vi "MOSFET Test.vi"() -> ()   [LabVIEW 2017]
uses:
  <instrlib>/Keithley 2600 Series/Public/Channel.ctl
  <instrlib>/Keithley 2600 Series/Keithley 2600 Series.lvlib
panel:
  in  "stop":bool
  in  "Tab Control":T1(tab)
  in  "GateCluster DFC":T2={"Gate channel DFC"=0, "Operation Mode"=0, "GateStart DFC"=0.0, "GateStopDFC"=0.0, "GateStepDFC"=1.0, "GateComp DFC"=0.1, "GateStartUnit DFC"=1, "GateStopUnit DFC "=1, "GateStepUnit DFC"=1, "GateComplUnit DFC"=2} {"GateComplUnit DFC" items=["μA", "mA", "A"]; "GateStepUnit DFC" items=["mV", "V"]; "GateStopUnit DFC" items=["mV", "V"]; "GateStartUnit DFC" items=["mV", "V"]; "Gate channel DFC" items=["Channel A", "Channel B"]; "GateComp DFC" min=0.001 max=10.0 step=0.001; "GateStepDFC" min=-200.0 max=200.0 step=1.0 format="%#.3f"; "GateStopDFC" min=-200.0 max=200.0 step=1.0 format="%#.3f"; "GateStart DFC" min=-200.0 max=200.0 step=1.0 format="%#.3f"; "Operation Mode" items=["Voltage Step"]}
  in  "DrainCluster DFC":T3={"Drain "=0, "Operation Mode"=0, "DrainStart DFC"=0.0, "DrainStop DFC"=0.0, "DrainStep DFC"=1.0, "DrainComp DFC"=0.1, "DrainStartUnit DFC"=1, "DrainStopUnit  DFC"=1, "DrainStepUnit DFC"=1, "DrainCompUnit DFC"=2, "DrainDelayUnit DFC"=0, "DrainDelay DFC"=1.0} {"DrainDelay DFC" min=1.0 max=6000.0 step=1.0 format="%#.3f"; "DrainDelayUnit DFC" items=["ms", "s"]; "DrainCompUnit DFC" items=["μA", "mA", "A"]; "DrainStepUnit DFC" items=["mV", "V"]; "DrainStopUnit  DFC" items=["mV", "V"]; "DrainStartUnit DFC" items=["mV", "V"]; "Drain" items=["Channel A", "Channel B"]; "DrainComp DFC" min=0.1 max=1.0 step=0.001 format="%#.3f"; "DrainStep DFC" min=-200.0 max=200.0 step=1.0 format="%#.3f"; "DrainStop DFC" min=-200.0 max=200.0 step=1.0 format="%#.3f"; "DrainStart DFC" min=-200.0 max=200.0 step=1.0 format="%#.3f"; "Operation Mode" items=["Voltage Linear Sweep"]}
  out "Chart DFC":cluster{dbl[], dbl[]}[](graph)
  out "Sheet DFC":string[][](table) caption="Sheet"
  in  "GateCluster TV":T4={"Gate CHTV"=0, "Operation Mode"=0, "Start GateTV"=0.0, "Stop GateTV"=0.0, "Step GateTV"=0.0, "Comp GateTV"=0.0, "StartUnit GateTV"=1, "StopUnit GateTV"=1, "StepUnit GateTV"=1, "CompUnit GateTV"=2} {"CompUnit GateTV" items=["μA", "mA", "A"]; "StepUnit GateTV" items=["mV", "V"]; "StopUnit GateTV" items=["mV", "V"]; "StartUnit GateTV" items=["mV", "V"]; "Gate CHTV" items=["Channel A", "Channel B"]; "Operation Mode" items=["None", "Voltage Step", "Voltage bias "]}
  in  "DrainClusterTV":T5={"Drain CHTV"=0, "Operation Mode"=0, "Start DrainTV"=0.0, "Stop DrainTV"=0.0, "Step DrainTV"=0.0, "Comp DrainTV"=0.0, "StartUnit DrainTV"=1, "StopUnit DrainTV"=1, "StepUnit DrainTV"=1, "CompUnit DrainTV"=2} {"CompUnit DrainTV" items=["μA", "mA", "A"]; "StepUnit DrainTV" items=["mV", "V"]; "StopUnit DrainTV" items=["mV", "V"]; "StartUnit DrainTV" items=["mV", "V"]; "Drain CHTV" items=["Channel A", "Channel B"]; "Operation Mode" items=["None", "Voltage Step", ""]}
  out "Chart TV":cluster{dbl[], dbl[]}[](graph)
  out "Sheet TV":string[][](table) caption="Sheet"
  in  "GateCluster GL":T6={"Gate CHGL"=0, "Operation Mode"=0, "Start GateGL"=0.0, "Stop GateGL"=0.0, "Step GateGL"=0.0, "Comp GateGL"=0.0, "StartUnit GateGL"=1, "StopUnit GateGL"=1, "StepUnit GateGL"=1, "CompUnit GateGL"=2, "GateDelayUnit GL"=0, "GateDelay GL"=1.0} {"GateDelay GL" min=1.0 max=6000.0 step=1.0 format="%#.3f"; "GateDelayUnit GL" items=["ms", "s"]; "CompUnit GateGL" items=["μA", "mA", "A"]; "StepUnit GateGL" items=["mV", "V"]; "StopUnit GateGL" items=["mV", "V"]; "StartUnit GateGL" items=["mV", "V"]; "Gate CHGL" items=["Channel A", "Channel B"]; "Operation Mode" items=["Voltage Sweep"]}
  out "Chart GL":cluster{dbl[], dbl[]}[](graph)
  out "Sheet GL":string[][](table) caption="Sheet"
  in  "GateCluster Trans":T7={"G channeTR"=0, "Operation Mode"=0, "Start  GateTR"=0.0, "Stop GateTR"=0.0, "Step GateTR"=0.0, "Comp GateTR"=0.0, "StartUnit GateTR"=1, "StopUnit GateTR"=1, "StepUnit GateTR"=1, "CompUnit GateTR"=2, "GateDelayUnit TR"=0, "GateDelayTR"=1.0} {"GateDelayTR" min=1.0 max=6000.0 step=1.0 format="%#.3f"; "GateDelayUnit TR" items=["ms", "s"]; "CompUnit GateTR" items=["μA", "mA", "A"]; "StepUnit GateTR" items=["mV", "V"]; "StopUnit GateTR" items=["mV", "V"]; "StartUnit GateTR" items=["mV", "V"]; "G channeTR" items=["Channel A", "Channel B"]; "Operation Mode" items=["Voltage Step"]}
  in  "DrainCluster Trans":T8={"D channelTR"=0, "Operation Mode"=0, "Start DrainTR"=0.0, "Comp DrainTR"=0.0, "StartUnit DrainTR"=1, "CompUnit DrainTR"=2} {"CompUnit DrainTR" items=["μA", "mA", "A"]; "StartUnit DrainTR" items=["mV", "V"]; "D channelTR" items=["Channel A", "Channel B"]; "Operation Mode" items=["Voltage Bias"]}
  out "Chart TR":cluster{dbl[], dbl[]}[](graph)
  out "Sheet TR":string[][](table) caption="Sheet"
  in  "Save Button":bool
  in  "Stop Button":bool
  in  "OK Button":bool
  in  "Series 2600B":u16(ring)=5 items=["2602B  40V, 10A,100fA", "2604B  40V, 10A,100fA", "2612B  200V, 10A,100fA", "2614B  200V, 10A,100fA", "2634B  200V, 10A,1fA", "2636B  200V, 10A,0.1fA"]
  # "PRCBE  2600B -MOSFET Test"
  # "V"
  # "V"
  # "V"
  # "A"
  # "V"
  # "V"
  # "V"
  # "A"
  # "V"
  # "V"
  # "V"
  # "A"
  # "V"
  # "V"
  # "V"
  # "A"
  # "V"
  # "V"
  # "V"
  # "A"
  # "V"
  # "V"
  # "V"
  # "A"
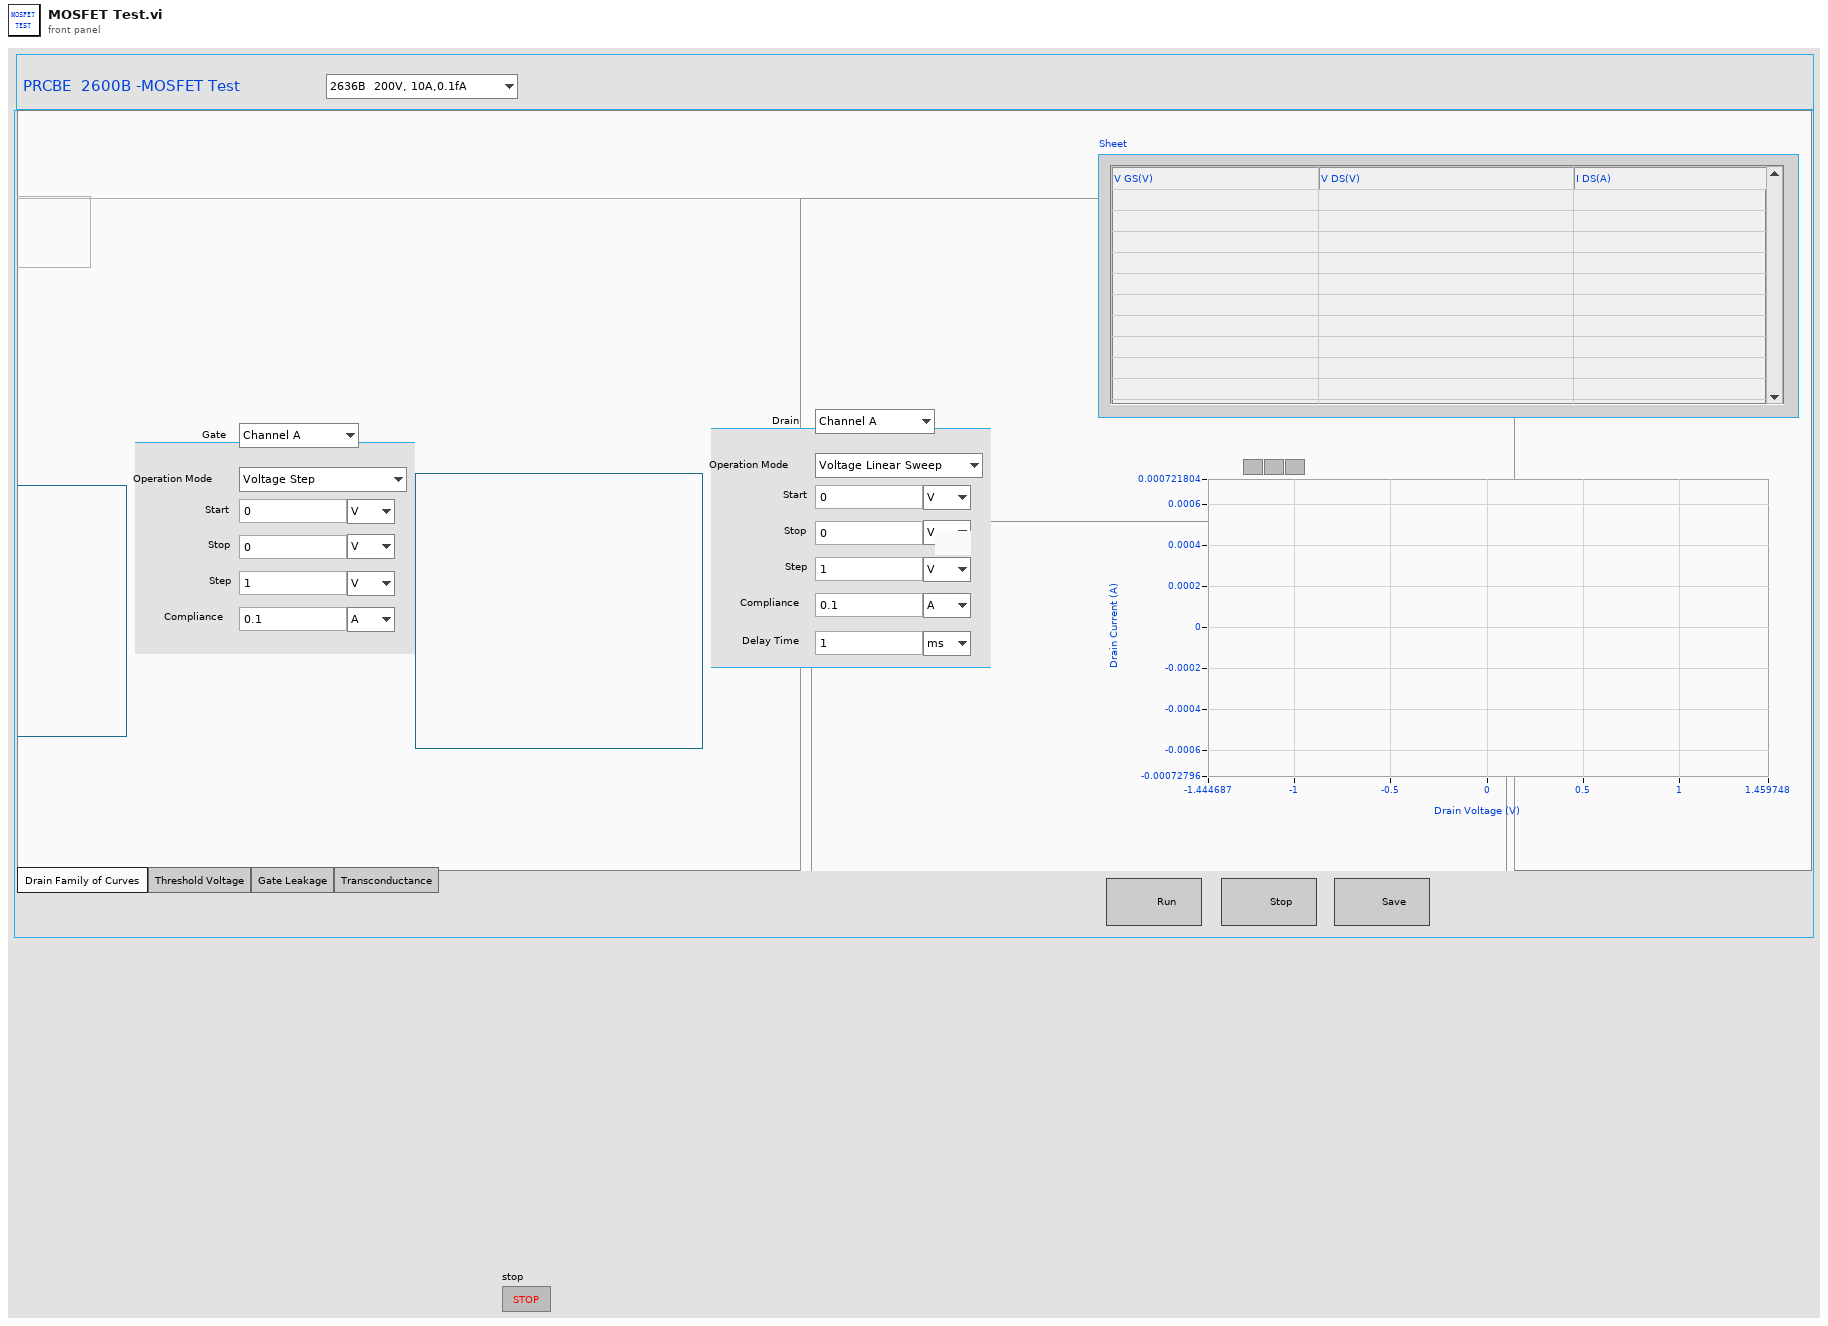
[diagram p1: front panel]
types:
  T1 = enum32{"Drain Family of Curves ", "Threshold Voltage", "Gate Leakage", "Transconductance"}
  T2 = cluster{"Gate channel DFC":u16, "Operation Mode":u16, "GateStart DFC":dbl, "GateStopDFC":dbl, "GateStepDFC":dbl, "GateComp DFC":dbl, "GateStartUnit DFC":u16, "GateStopUnit DFC ":u16, "GateStepUnit DFC":u16, "GateComplUnit DFC":u16}
  T3 = cluster{"Drain ":u16, "Operation Mode":u16, "DrainStart DFC":dbl, "DrainStop DFC":dbl, "DrainStep DFC":dbl, "DrainComp DFC":dbl, "DrainStartUnit DFC":u16, "DrainStopUnit  DFC":u16, "DrainStepUnit DFC":u16, "DrainCompUnit DFC":u16, "DrainDelayUnit DFC":u16, "DrainDelay DFC":dbl}
  T4 = cluster{"Gate CHTV":u16, "Operation Mode":u16, "Start GateTV":dbl, "Stop GateTV":dbl, "Step GateTV":dbl, "Comp GateTV":dbl, "StartUnit GateTV":u16, "StopUnit GateTV":u16, "StepUnit GateTV":u16, "CompUnit GateTV":u16}
  T5 = cluster{"Drain CHTV":u16, "Operation Mode":u16, "Start DrainTV":dbl, "Stop DrainTV":dbl, "Step DrainTV":dbl, "Comp DrainTV":dbl, "StartUnit DrainTV":u16, "StopUnit DrainTV":u16, "StepUnit DrainTV":u16, "CompUnit DrainTV":u16}
  T6 = cluster{"Gate CHGL":u16, "Operation Mode":u16, "Start GateGL":dbl, "Stop GateGL":dbl, "Step GateGL":dbl, "Comp GateGL":dbl, "StartUnit GateGL":u16, "StopUnit GateGL":u16, "StepUnit GateGL":u16, "CompUnit GateGL":u16, "GateDelayUnit GL":u16, "GateDelay GL":dbl}
  T7 = cluster{"G channeTR":u16, "Operation Mode":u16, "Start  GateTR":dbl, "Stop GateTR":dbl, "Step GateTR":dbl, "Comp GateTR":dbl, "StartUnit GateTR":u16, "StopUnit GateTR":u16, "StepUnit GateTR":u16, "CompUnit GateTR":u16, "GateDelayUnit TR":u16, "GateDelayTR":dbl}
  T8 = cluster{"D channelTR":u16, "Operation Mode":u16, "Start DrainTR":dbl, "Comp DrainTR":dbl, "StartUnit DrainTR":u16, "CompUnit DrainTR":u16}
  T9 = cluster{"Drain ":u16, "Operation Mode":u16, "DrainStart DFC":dbl, "DrainStop DFC":dbl, "DrainStep DFC":dbl, "DrainComp DFC":dbl, "DrainStartUnit DFC":u16, "DrainStopUnit  DFC":u16, "DrainStepUnit DFC":u16, "DrainCompUnit DFC":u16, "DrainDelay DFC":dbl, "DrainDelayUnit DFC":u16}
  T10 = typedef "Keithley 2600 Series.lvlib/Channel.ctl" = enum32{"Channel A", "Channel B"}
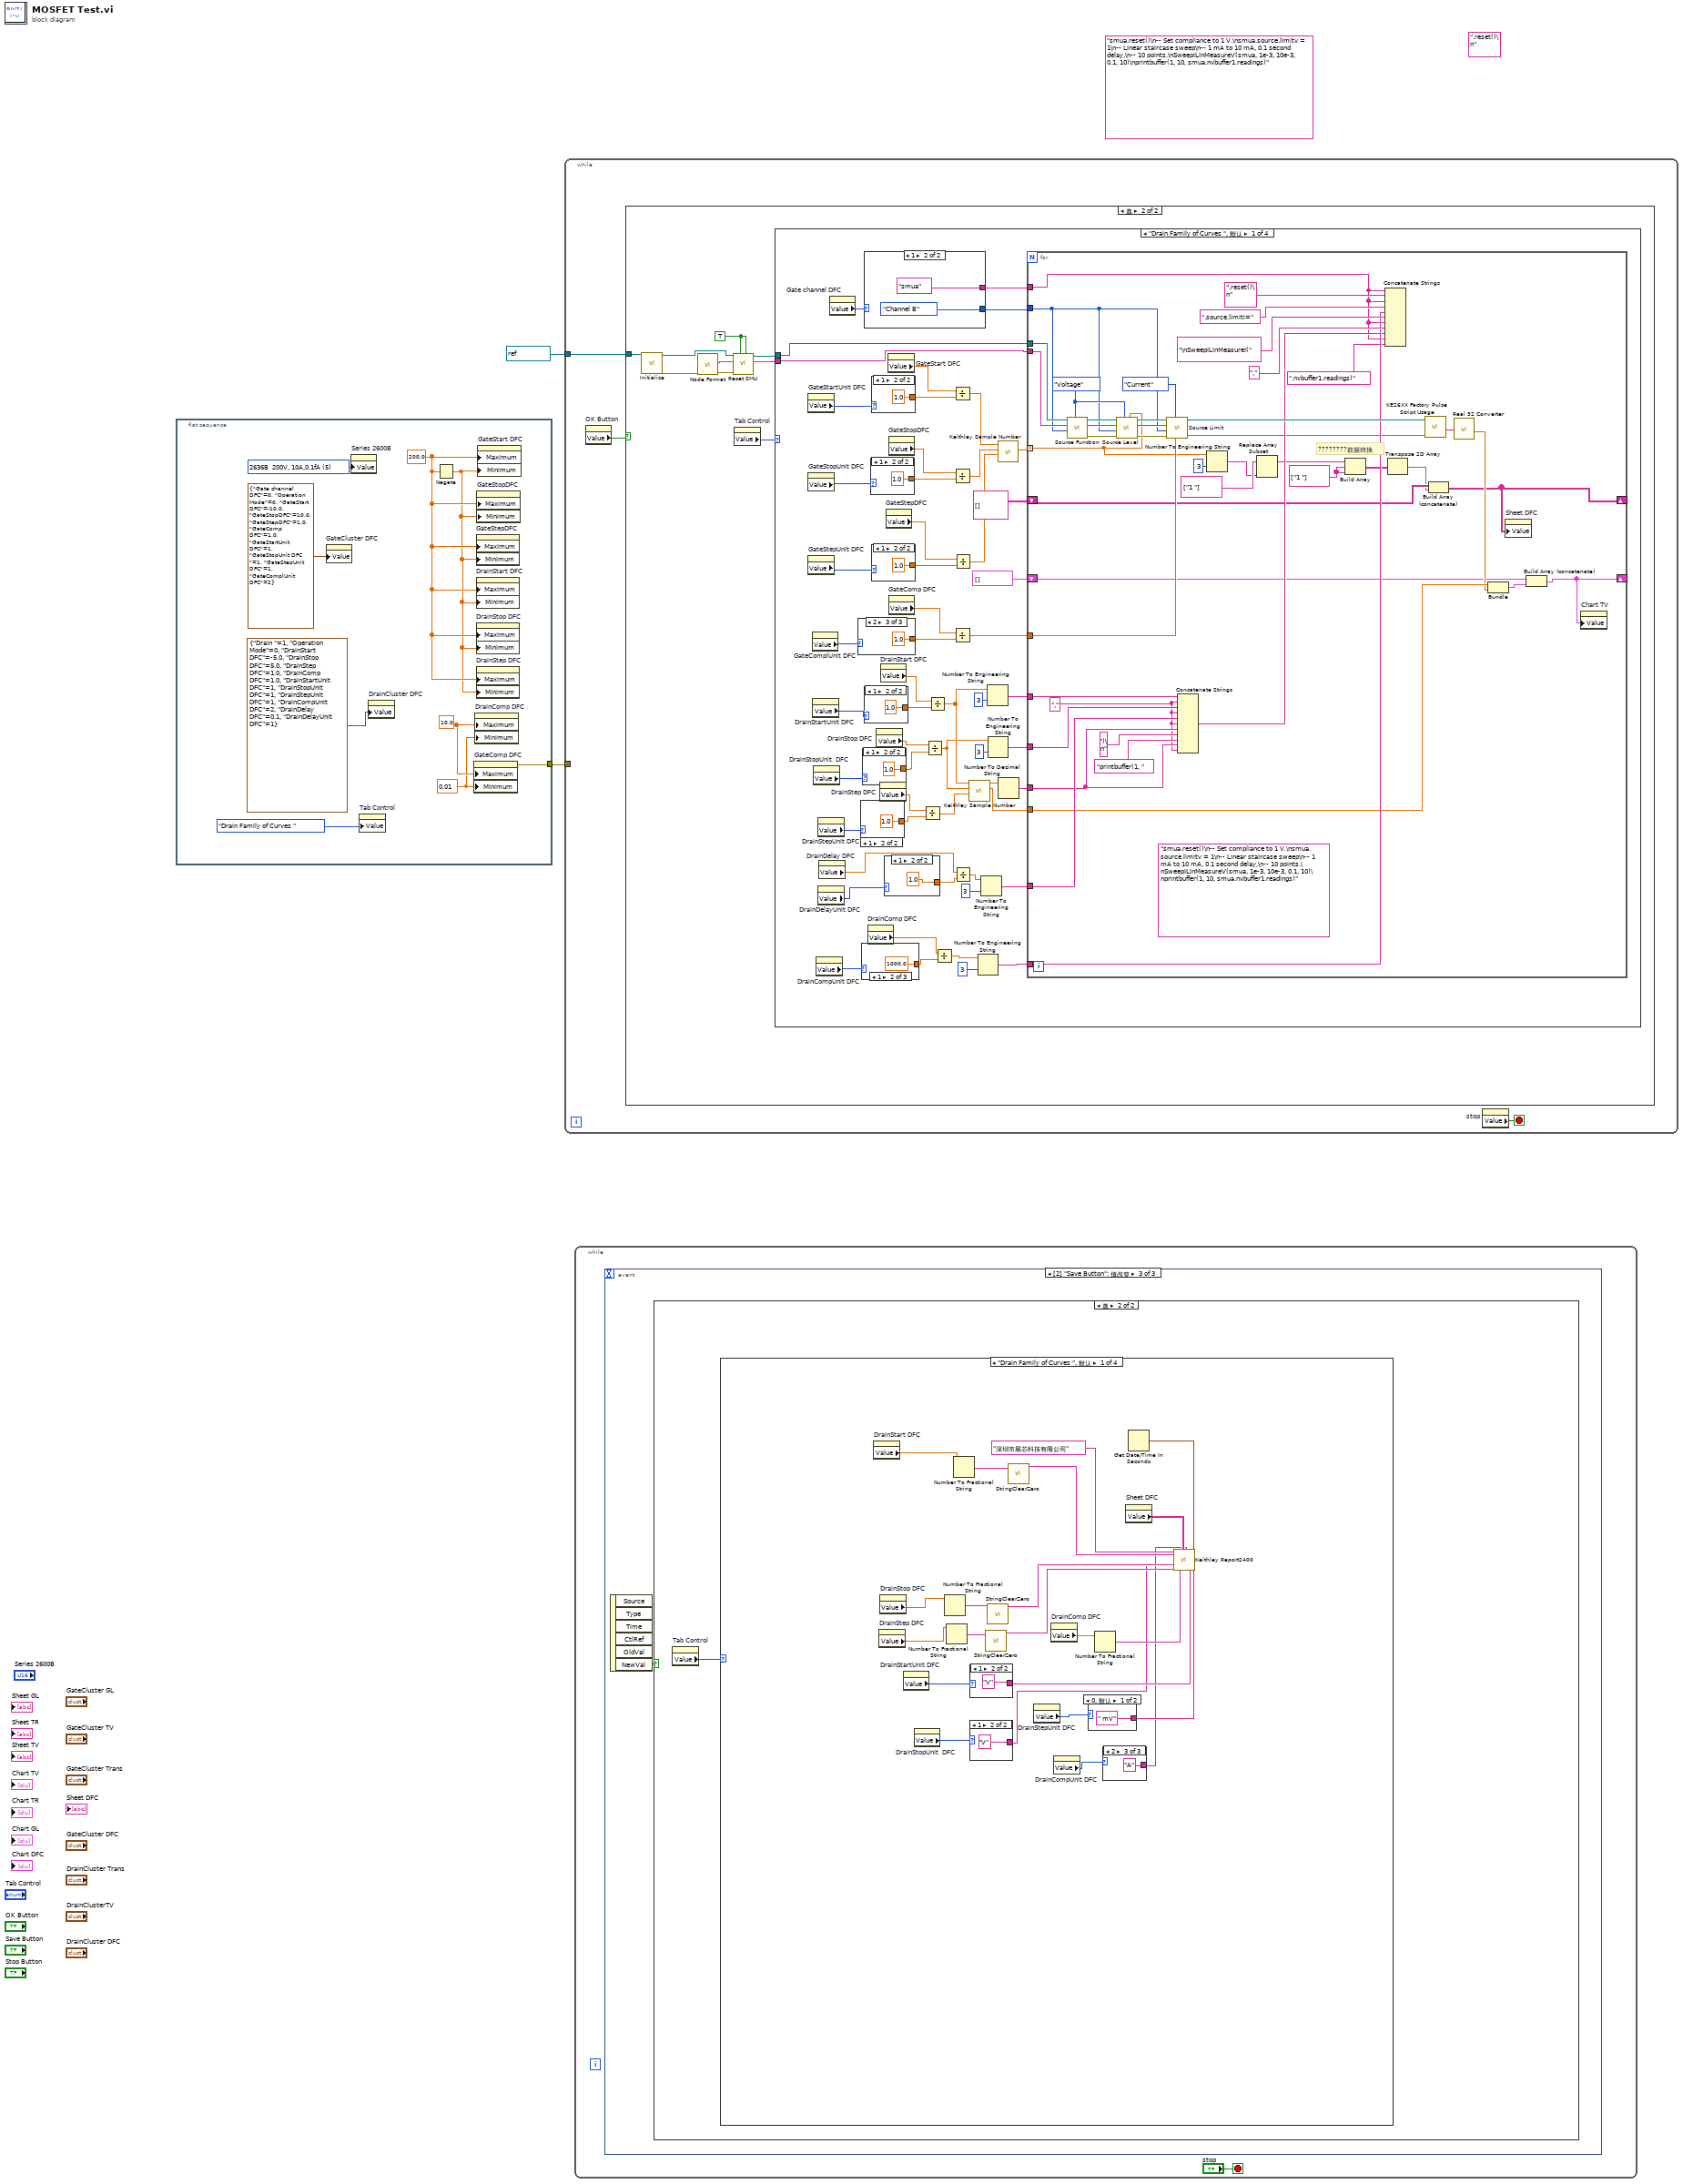
[diagram p0: block diagram]
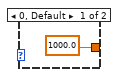
[diagram p3: hidden frame]
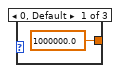
[diagram p4: hidden frame]
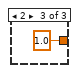
[diagram p5: hidden frame]
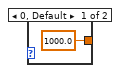
[diagram p6: hidden frame]
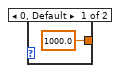
[diagram p7: hidden frame]
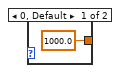
[diagram p8: hidden frame]
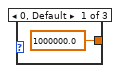
[diagram p9: hidden frame]
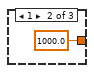
[diagram p10: hidden frame]
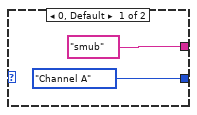
[diagram p11: hidden frame]
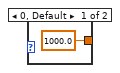
[diagram p12: hidden frame]
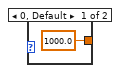
[diagram p13: hidden frame]
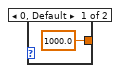
[diagram p14: hidden frame]
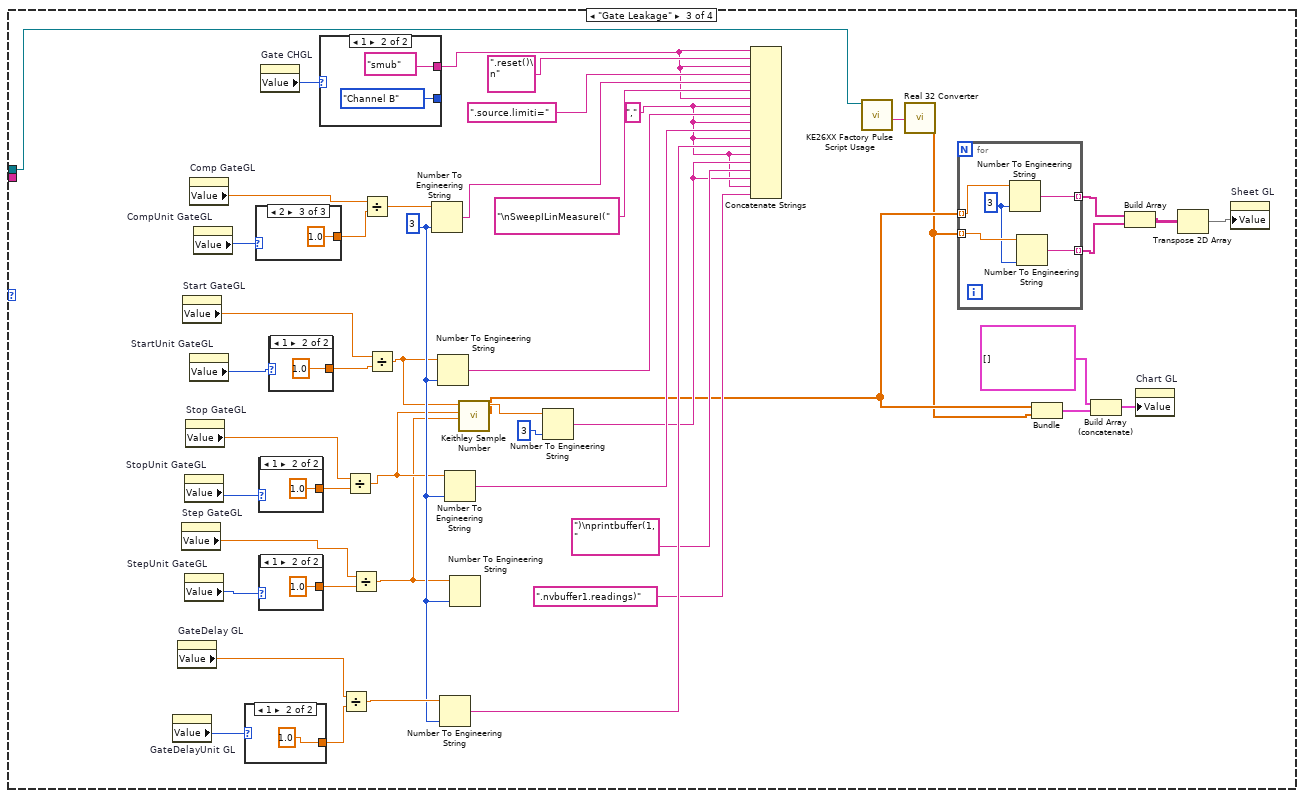
[diagram p16: hidden frame]
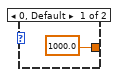
[diagram p17: hidden frame]
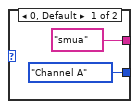
[diagram p18: hidden frame]
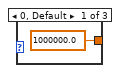
[diagram p19: hidden frame]
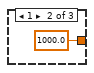
[diagram p20: hidden frame]
diagram:
  (unwired) ".reset()\n" ("string")
  (unwired) "smua.reset()\n-- Set compliance to 1 V.\nsmua.source.limitv = 1\n-- Linear staircase sweep\n-- 1 mA to 10 mA, 0.1 second delay,\n-- 10 points.\nSweepILinMeasureV(smua, 1e-3, 10e-3, 0.1, 10)\nprintbuffer(1, 10, smua.nvbuffer1.readings)" ("Script")
  n1 = flat-sequence {
    tunnel: [w3] -> w1
    frame #0 {
      w6 = 0.01 ("Data Entry Limits:Minimum")
      w7 = 10.0 ("Data Entry Limits:Maximum")
      w9 = 200.0 ("Data Entry Limits:Maximum")
      w11 = u16 5 items=["2602B  40V, 10A,100fA", "2604B  40V, 10A,100fA", "2612B  200V, 10A,100fA", "2614B  200V, 10A,100fA", "2634B  200V, 10A,1fA", "2636B  200V, 10A,0.1fA"] ("Series 2600B")
      n2 = property on="GateCluster DFC" class="Clust (严格)"("Value"=T2 {"Gate channel DFC"=0, "Operation Mode"=0, "GateStart DFC"=-10.0, "GateStopDFC"=10.0, "GateStepDFC"=1.0, "GateComp DFC"=1.0, "GateStartUnit DFC"=1, "GateStopUnit DFC "=1, "GateStepUnit DFC"=1, "GateComplUnit DFC"=2} ("GateCluster DFC")) -> ()  [unwired: 2 in, 2 out]
      n3 = property on="Series 2600B" class="Ring (严格)"("Value"=w11) -> ()  [unwired: 2 in, 2 out]
      n4 = property on="Tab Control" class="TabCtl (严格)"("Value"=T1."Drain Family of Curves " ("Tab Control")) -> ()  [unwired: 2 in, 2 out]
      n5 = property on="DrainCluster DFC" class="Clust (严格)"("Value"=T9 {"Drain "=1, "Operation Mode"=0, "DrainStart DFC"=-5.0, "DrainStop DFC"=5.0, "DrainStep DFC"=1.0, "DrainComp DFC"=1.0, "DrainStartUnit DFC"=1, "DrainStopUnit  DFC"=1, "DrainStepUnit DFC"=1, "DrainCompUnit DFC"=2, "DrainDelay DFC"=0.1, "DrainDelayUnit DFC"=1} ("DrainCluster DFC")) -> ()  [unwired: 2 in, 2 out]
      n6 = Negate(x=w9) -> (-x=w8:dbl)
      n7 = property on="GateComp DFC" class="DigNum (严格)"("Maximum"=w7, "Minimum"=w6) -> (error out=w3:errorcluster)  [unwired: 2 in, 1 out]
      n8 = property on="DrainComp DFC" class="DigNum (严格)"("Maximum"=w7, "Minimum"=w6) -> ()  [unwired: 2 in, 2 out]
      n9 = property on="GateStepDFC" class="DigNum (严格)"("Maximum"=w9, "Minimum"=w8) -> ()  [unwired: 2 in, 2 out]
      n10 = property on="DrainStart DFC" class="DigNum (严格)"("Maximum"=w9, "Minimum"=w8) -> ()  [unwired: 2 in, 2 out]
      n11 = property on="DrainStop DFC" class="DigNum (严格)"("Maximum"=w9, "Minimum"=w8) -> ()  [unwired: 2 in, 2 out]
      n12 = property on="DrainStep DFC" class="DigNum (严格)"("Maximum"=w9, "Minimum"=w8) -> ()  [unwired: 2 in, 2 out]
      n13 = property on="GateStopDFC" class="DigNum (严格)"("Maximum"=w9, "Minimum"=w8) -> ()  [unwired: 2 in, 2 out]
      n14 = property on="GateStart DFC" class="DigNum (严格)"("Maximum"=w9, "Minimum"=w8) -> ()  [unwired: 2 in, 2 out]
    }
  }
  n15 = while {
    tunnel: refnum<visa-resource-name> "COM1" ("VISA resource name") -> [w12]
    tunnel: w1 -> [_]
    stop <- w14 stop-if-true
    n16 = property on="OK Button" class="Bool (严格)"() -> ("Value"=w13:bool)  [unwired: 2 in, 2 out]
    n17 = case shown="真" w13 {
      tunnel: w12 -> [_ w22]
      frame False {
      }
      frame True {
        w17 = TRUE ("SMU A (No)")
        n18 = call <instrlib>:"Initialize.vi"("VISA resource name"=w22) -> ("error out"=w21:errorcluster, "VISA resource name out"=w20:refnum<visa-resource-name>)  [unwired: 4 in, 5 out]
        n19 = call <instrlib>:"Node Format.vi"("error in"=w21) -> ("error out"=w18:errorcluster, "Formatted Node"=w19:string)  [unwired: 1 in, 8 out]
        n20 = call <instrlib>:"Reset SMU.vi"("SMU B (No)"=w17, "SMU A (No)"=w17, "error in (no error)"=w18, "Node In"=w19, "VISA resource name"=w20) -> ("Node Out"=w15:string, "VISA resource name out"=w16:refnum<visa-resource-name>)  [unwired: 5 out]
        n21 = property on="Tab Control" class="TabCtl (严格)"() -> ("Value"=w23:T1)  [unwired: 2 in, 2 out]
        n22 = case shown="\"Drain Family of Curves \", 默认" w23 {
          tunnel: w16 -> [w65 _ w176 w227]
          tunnel: w15 -> [w63 _ _ w223]
          frame "Drain Family of Curves ", Default {
            n23 = property on="GateStartUnit DFC" class="Ring (严格)"() -> ("Value"=w78:u16)  [unwired: 2 in, 2 out]
            n24 = property on="GateStopUnit DFC" class="Ring (严格)"() -> ("Value"=w75:u16)  [unwired: 2 in, 2 out]
            n25 = property on="GateStepUnit DFC" class="Ring (严格)"() -> ("Value"=w72:u16)  [unwired: 2 in, 2 out]
            n26 = property on="GateComplUnit DFC" class="Ring (严格)"() -> ("Value"=w61:u16)  [unwired: 2 in, 2 out]
            n27 = property on="DrainStartUnit DFC" class="Ring (严格)"() -> ("Value"=w55:u16)  [unwired: 2 in, 2 out]
            n28 = property on="DrainStopUnit  DFC" class="Ring (严格)"() -> ("Value"=w52:u16)  [unwired: 2 in, 2 out]
            n29 = property on="DrainCompUnit DFC" class="Ring (严格)"() -> ("Value"=w43:u16)  [unwired: 2 in, 2 out]
            n30 = property on="DrainStepUnit DFC" class="Ring (严格)"() -> ("Value"=w51:u16)  [unwired: 2 in, 2 out]
            n31 = property on="DrainDelayUnit DFC" class="Ring (严格)"() -> ("Value"=w29:u16)  [unwired: 2 in, 2 out]
            n32 = property on="DrainDelay DFC" class="DigNum (严格)"() -> ("Value"=w33:dbl)  [unwired: 2 in, 2 out]
            n33 = property on="Gate channel DFC" class="Ring (严格)"() -> ("Value"=w64:u16)  [unwired: 2 in, 2 out]
            n34 = case shown="2" w61 {
              tunnel: [1000000.0 ("Value") 1000.0 ("Value") 1.0 ("Value")] -> w60
              frame 0, Default {
              }
              frame 1 {
              }
              frame 2 {
              }
            }
            n35 = case shown="1" w51 {
              tunnel: [1000.0 ("Value") 1.0 ("Value")] -> w48
              frame 0, Default {
              }
              frame 1 {
              }
            }
            n36 = case shown="1" w43 {
              tunnel: [1000000.0 ("Value") 1000.0 ("Value") 1.0 ("Value")] -> w45
              frame 0, Default {
              }
              frame 1 {
              }
              frame 2 {
              }
            }
            n37 = case shown="1" w52 {
              tunnel: [1000.0 ("Value") 1.0 ("Value")] -> w49
              frame 0, Default {
              }
              frame 1 {
              }
            }
            n38 = case shown="1" w64 {
              tunnel: [Channel."Channel A" ("Channel (Channel A)") Channel."Channel B" ("Channel (Channel A)")] -> w62
              tunnel: ["smub" ("Script") "smua" ("Script")] -> w57
              frame 0, Default {
              }
              frame 1 {
              }
            }
            n39 = case shown="1" w55 {
              tunnel: [1000.0 ("Value") 1.0 ("Value")] -> w56
              frame 0, Default {
              }
              frame 1 {
              }
            }
            n40 = property on="DrainComp DFC" class="DigNum (严格)"() -> ("Value"=w44:dbl)  [unwired: 2 in, 2 out]
            n41 = case shown="1" w75 {
              tunnel: [1000.0 ("Value") 1.0 ("Value")] -> w73
              frame 0, Default {
              }
              frame 1 {
              }
            }
            n42 = case shown="1" w78 {
              tunnel: [1000.0 ("Value") 1.0 ("Value")] -> w77
              frame 0, Default {
              }
              frame 1 {
              }
            }
            n43 = case shown="1" w72 {
              tunnel: [1000.0 ("Value") 1.0 ("Value")] -> w71
              frame 0, Default {
              }
              frame 1 {
              }
            }
            n44 = property on="DrainStop DFC" class="DigNum (严格)"() -> ("Value"=w53:dbl)  [unwired: 2 in, 2 out]
            n45 = property on="DrainStep DFC" class="DigNum (严格)"() -> ("Value"=w50:dbl)  [unwired: 2 in, 2 out]
            n46 = property on="DrainStart DFC" class="DigNum (严格)"() -> ("Value"=w54:dbl)  [unwired: 2 in, 2 out]
            n47 = case shown="1" w29 {
              tunnel: [1000.0 ("Value") 1.0 ("Value")] -> w32
              frame 0, Default {
              }
              frame 1 {
              }
            }
            n48 = property on="GateStepDFC" class="DigNum (严格)"() -> ("Value"=w70:dbl)  [unwired: 2 in, 2 out]
            n49 = property on="GateStart DFC" class="DigNum (严格)"() -> ("Value"=w76:dbl)  [unwired: 2 in, 2 out]
            n50 = property on="GateStopDFC" class="DigNum (严格)"() -> ("Value"=w74:dbl)  [unwired: 2 in, 2 out]
            n51 = property on="GateComp DFC" class="DigNum (严格)"() -> ("Value"=w59:dbl)  [unwired: 2 in, 2 out]
            n52 = Divide(x=w50, y=w48) -> (x/y=w47:dbl)
            n53 = Divide(x=w53, y=w49) -> (x/y=w27:dbl)
            n54 = Divide(x=w54, y=w56) -> (x/y=w37:dbl)
            n55 = Divide(x=w44, y=w45) -> (x/y=w41:dbl)
            n56 = Divide(x=w76, y=w77) -> (x/y=w69:dbl)
            n57 = Divide(x=w74, y=w73) -> (x/y=w68:dbl)
            n58 = Divide(x=w59, y=w60) -> (x/y=w58:dbl)
            n59 = Divide(x=w70, y=w71) -> (x/y=w67:dbl)
            n60 = Divide(x=w33, y=w32) -> (x/y=w30:dbl)
            n61 = call "Keithley Sample Number.vi"("Step"=w47, "Stop"=w27, "Start"=w37) -> ("Array"=w26:dbl[], "pointnumber"=w46:dbl)  [unwired: 7 in]
            n62 = Number To Engineering String(2:i16 3 ("precision (6)"), 4:w41) -> (0:w40:string)  [unwired: 2 in]
            n63 = Number To Engineering String(2:i16 3 ("precision (6)"), 4:w30) -> (0:w28:string)  [unwired: 2 in]
            n64 = Number To Engineering String(2:i16 3 ("precision (6)"), 4:w37) -> (0:w34:string)  [unwired: 2 in]
            n65 = Number To Engineering String(2:i16 3 ("precision (6)"), 4:w27) -> (0:w35:string)  [unwired: 2 in]
            n66 = call "Keithley Sample Number.vi"("Step"=w67, "Stop"=w68, "Start"=w69) -> ("Array"=w66:dbl[])  [unwired: 7 in, 1 out]
            n67 = Number To Decimal String(number=w46) -> (decimal integer string=w39:string)  [unwired: 1 in]
            n68 = for {
              tunnel: w66 -> [w105] mode=indexing
              tunnel: w65 -> [w137]
              tunnel: w63 -> [w136]
              tunnel: w62 -> [w132]
              tunnel: w58 -> [w127]
              tunnel: w57 -> [w116]
              tunnel: w40 -> [w124]
              tunnel: w39 -> [w118]
              tunnel: w35 -> [w122]
              tunnel: w34 -> [w123]
              tunnel: w28 -> [w121]
              tunnel: w26 -> [w111]
              shift-right: [w107] -> _
              shift-left: cluster{dbl[], dbl[]}[] [] ("Chart TV") -> [w109]
              shift-right: [w97] -> _
              shift-left: string[][] [] ("Sheet DFC") -> [w103]
              w104 = string[] ["1 "]
              (unwired) "smua.reset()\n-- Set compliance to 1 V.\nsmua.source.limitv = 1\n-- Linear staircase sweep\n-- 1 mA to 10 mA, 0.1 second delay,\n-- 10 points.\nSweepILinMeasureV(smua, 1e-3, 10e-3, 0.1, 10)\nprintbuffer(1, 10, smua.nvbuffer1.readings)" ("Script")
              w115 = "," ("string")
              w135 = enum32{"Current", "Voltage"}."Voltage" ("Function (Current)")
              # "????????数据转换"
              n69 = call <instrlib>:"Source Function.vi"("Function (Current)"=w135, "Channel (Channel A)"=w132, "Node In"=w136, "VISA resource name"=w137) -> ("error out"=w134:errorcluster, "Node Out"=w138:string, "VISA resource name out"=w139:refnum<visa-resource-name>)  [unwired: 1 in, 4 out]
              n70 = call <instrlib>:"Source Level.vi"("Level (0.000)"=w105, "Function (Current)"=w135, "error in (no error)"=w134, "Channel (Channel A)"=w132, "Node In"=w138, "VISA resource name"=w139) -> ("error out"=w133:errorcluster, "Node Out"=w141:string, "VISA resource name out"=w140:refnum<visa-resource-name>)  [unwired: 3 out]
              n71 = call <instrlib>:"Source Limit.vi"("Limit (0.000)"=w127, "Function (Current)"=enum32{"Current", "Voltage"}."Current", "error in (no error)"=w133, "Channel (Channel A)"=w132, "Node In"=w141, "VISA resource name"=w140) -> ("error out"=w113:errorcluster, "VISA resource name out"=w130:refnum<visa-resource-name>)  [unwired: 4 out]
              n72 = Concatenate Strings(w123, w115, w122, w115, w121, w115, w118, ")\n" ("string"), "printbuffer(1, " ("string"), w118, w115) -> (w117:string)
              n73 = Number To Engineering String(2:i16 3 ("precision (6)"), 4:w105) -> (0:w101:string)  [unwired: 2 in]
              n74 = Replace Array Subset(array=string[] ["1 "], new element=w101) -> (w100:string[])  [unwired: 1 in]
              n75 = Build Array(w100, w104, w104) -> (w99:string[][])
              n76 = Concatenate Strings(w116, ".reset()\n" ("string"), w116, ".source.limiti=" ("string"), w124, "\nSweepILinMeasureI(" ("string"), w116, "," ("string"), w117, w116, ".nvbuffer1.readings)" ("string")) -> ()  [unwired: 1 out]
              n77 = Transpose 2D Array(2D array=w99) -> (transposed array=w98:string[][])
              n78 = call <instrlib>:"KE26XX Factory Pulse Script Usage.vi"("error in"=w113, "VISA resource name"=w130) -> ("Buffer Data"=w112:string)  [unwired: 8 in, 1 out]
              n79 = Build Array (concatenate)(w103, w98) -> (w97:string[][])
              n80 = call <instrlib>:"Real 32 Converter.vi"("Data In"=w112) -> ("Data Array Out"=w110:sgl[])  [unwired: 10 in]
              n81 = Bundle("Array"=w111, "Data Array Out"=w110) -> (w108:cluster{"Array":dbl[], "Data Array Out":sgl[]})  [unwired: 1 in]
              n82 = property on="Sheet DFC" class="Tbl (严格)"("Value"=w97) -> ()  [unwired: 2 in, 2 out]
              n83 = Build Array (concatenate)(w109, w108) -> (w107:cluster{"Array":dbl[], "Data Array Out":dbl[]}[])
              n84 = property on="Chart TV" class="XYGraph (严格)"("Value"=w107) -> ()  [unwired: 2 in, 2 out]
            }
          }
          frame "Threshold Voltage" {
          }
          frame "Gate Leakage" {
            w158 = "," ("string")
            w174 = i16 3 ("precision (6)")
            n85 = property on="GateDelayUnit GL" class="Ring (严格)"() -> ("Value"=w173:u16)  [unwired: 2 in, 2 out]
            n86 = property on="GateDelay GL" class="DigNum (严格)"() -> ("Value"=w171:dbl)  [unwired: 2 in, 2 out]
            n87 = property on="Step GateGL" class="DigNum (严格)"() -> ("Value"=w187:dbl)  [unwired: 2 in, 2 out]
            n88 = property on="Start GateGL" class="DigNum (严格)"() -> ("Value"=w193:dbl)  [unwired: 2 in, 2 out]
            n89 = property on="StopUnit GateGL" class="Ring (严格)"() -> ("Value"=w189:u16)  [unwired: 2 in, 2 out]
            n90 = property on="StepUnit GateGL" class="Ring (严格)"() -> ("Value"=w186:u16)  [unwired: 2 in, 2 out]
            n91 = property on="Stop GateGL" class="DigNum (严格)"() -> ("Value"=w190:dbl)  [unwired: 2 in, 2 out]
            n92 = property on="Comp GateGL" class="DigNum (严格)"() -> ("Value"=w184:dbl)  [unwired: 2 in, 2 out]
            n93 = property on="StartUnit GateGL" class="Ring (严格)"() -> ("Value"=w194:u16)  [unwired: 2 in, 2 out]
            n94 = property on="CompUnit GateGL" class="Ring (严格)"() -> ("Value"=w183:u16)  [unwired: 2 in, 2 out]
            n95 = case shown="1" w173 {
              tunnel: [1000.0 ("Value") 1.0 ("Value")] -> w172
              frame 0, Default {
              }
              frame 1 {
              }
            }
            n96 = case shown="2" w183 {
              tunnel: [1000000.0 ("Value") 1000.0 ("Value") 1.0 ("Value")] -> w185
              frame 0, Default {
              }
              frame 1 {
              }
              frame 2 {
              }
            }
            n97 = case shown="1" w189 {
              tunnel: [1000.0 ("Value") 1.0 ("Value")] -> w191
              frame 0, Default {
              }
              frame 1 {
              }
            }
            n98 = case shown="1" w186 {
              tunnel: [1000.0 ("Value") 1.0 ("Value")] -> w188
              frame 0, Default {
              }
              frame 1 {
              }
            }
            n99 = property on="Gate CHGL" class="Ring (严格)"() -> ("Value"=w182:u16)  [unwired: 2 in, 2 out]
            n100 = case shown="1" w194 {
              tunnel: [1000.0 ("Value") 1.0 ("Value")] -> w192
              frame 0, Default {
              }
              frame 1 {
              }
            }
            n101 = case shown="1" w182 {
              tunnel: [Channel."Channel A" ("Channel (Channel A)") Channel."Channel B" ("Channel (Channel A)")] -> _
              tunnel: ["smua" ("Script") "smub" ("Script")] -> w166
              frame 0, Default {
              }
              frame 1 {
              }
            }
            n102 = Divide(x=w171, y=w172) -> (x/y=w175:dbl)
            n103 = Divide(x=w190, y=w191) -> (x/y=w169:dbl)
            n104 = Divide(x=w187, y=w188) -> (x/y=w168:dbl)
            n105 = Divide(x=w184, y=w185) -> (x/y=w178:dbl)
            n106 = Divide(x=w193, y=w192) -> (x/y=w170:dbl)
            n107 = Number To Engineering String(2:w174, 4:w178) -> (0:w177:string)  [unwired: 2 in]
            n108 = Number To Engineering String(2:w174, 4:w170) -> (0:w165:string)  [unwired: 2 in]
            n109 = Number To Engineering String(2:w174, 4:w175) -> (0:w163:string)  [unwired: 2 in]
            n110 = Number To Engineering String(2:w174, 4:w169) -> (0:w164:string)  [unwired: 2 in]
            n111 = Number To Engineering String(2:w174, 4:w168) -> ()  [unwired: 2 in, 1 out]
            n112 = call "Keithley Sample Number.vi"("Step"=w168, "Stop"=w169, "Start"=w170) -> ("Array"=w152:dbl[], "pointnumber"=w161:dbl)  [unwired: 7 in]
            n113 = Number To Engineering String(2:i16 3 ("precision (6)"), 4:w161) -> (0:w159:string)  [unwired: 2 in]
            n114 = Concatenate Strings(w166, ".reset()\n" ("string"), w166, ".source.limiti=" ("string"), w177, "\nSweepILinMeasureI(" ("string"), w166, w158, w165, w158, w164, w158, w163, w158, w159, ")\nprintbuffer(1, " ("string"), w159, w158, ".nvbuffer1.readings)" ("string")) -> ()  [unwired: 1 out]
            n115 = call <instrlib>:"KE26XX Factory Pulse Script Usage.vi"("VISA resource name"=w176) -> ("Buffer Data"=w181:string)  [unwired: 9 in, 1 out]
            n116 = call <instrlib>:"Real 32 Converter.vi"("Data In"=w181) -> ("Data Array Out"=w151:sgl[])  [unwired: 10 in]
            n117 = for {
              tunnel: w152 -> [w199] mode=indexing
              tunnel: w151 -> [w197] mode=indexing
              tunnel: [w198] -> w150 mode=indexing
              tunnel: [w195] -> w149 mode=indexing
              w196 = i16 3 ("precision (6)")
              n118 = Number To Engineering String(2:w196, 4:w199) -> (0:w198:string)  [unwired: 2 in]
              n119 = Number To Engineering String(2:w196, 4:w197) -> (0:w195:string)  [unwired: 2 in]
            }
            n120 = Bundle("Array"=w152, "Data Array Out"=w151) -> (w155:cluster{"Array":dbl[], "Data Array Out":sgl[]})  [unwired: 1 in]
            n121 = Build Array (concatenate)(cluster{dbl[], dbl[]}[] [] ("Chart GL"), w155) -> (w154:cluster{"Array":dbl[], "Data Array Out":dbl[]}[])
            n122 = Build Array(w150, w149) -> (w153:string[][])
            n123 = property on="Chart GL" class="XYGraph (严格)"("Value"=w154) -> ()  [unwired: 2 in, 2 out]
            n124 = Transpose 2D Array(2D array=w153) -> (transposed array=w148:string[][])
            n125 = property on="Sheet GL" class="Tbl (严格)"("Value"=w148) -> ()  [unwired: 2 in, 2 out]
          }
          frame "Transconductance" {
            w231 = enum32{"Current", "Voltage"}."Voltage" ("Function (Current)")
            w247 = "," ("string")
            w263 = i16 3 ("precision (6)")
            # "??/????数据转换确认"
            n126 = property on="GateDelayTR" class="DigNum (严格)"() -> ("Value"=w260:dbl)  [unwired: 2 in, 2 out]
            n127 = property on="GateDelayUnit TR" class="Ring (严格)"() -> ("Value"=w262:u16)  [unwired: 2 in, 2 out]
            n128 = property on="Step GateTR" class="DigNum (严格)"() -> ("Value"=w274:dbl)  [unwired: 2 in, 2 out]
            n129 = property on="Stop GateTR" class="DigNum (严格)"() -> ("Value"=w277:dbl)  [unwired: 2 in, 2 out]
            n130 = property on="StopUnit GateTR" class="Ring (严格)"() -> ("Value"=w276:u16)  [unwired: 2 in, 2 out]
            n131 = property on="StepUnit GateTR" class="Ring (严格)"() -> ("Value"=w273:u16)  [unwired: 2 in, 2 out]
            n132 = property on="StartUnit GateTR" class="Ring (严格)"() -> ("Value"=w281:u16)  [unwired: 2 in, 2 out]
            n133 = property on="Start  GateTR" class="DigNum (严格)"() -> ("Value"=w280:dbl)  [unwired: 2 in, 2 out]
            n134 = property on="Comp GateTR" class="DigNum (严格)"() -> ("Value"=w271:dbl)  [unwired: 2 in, 2 out]
            n135 = property on="CompUnit GateTR" class="Ring (严格)"() -> ("Value"=w270:u16)  [unwired: 2 in, 2 out]
            n136 = property on="CompUnit DrainTR" class="Ring (严格)"() -> ("Value"=w219:u16)  [unwired: 2 in, 2 out]
            n137 = property on="G channeTR" class="Ring (严格)"() -> ("Value"=w245:u16)  [unwired: 2 in, 2 out]
            n138 = property on="Comp DrainTR" class="DigNum (严格)"() -> ("Value"=w218:dbl)  [unwired: 2 in, 2 out]
            n139 = property on="StartUnit DrainTR" class="Ring (严格)"() -> ("Value"=w216:u16)  [unwired: 2 in, 2 out]
            n140 = property on="Start DrainTR" class="DigNum (严格)"() -> ("Value"=w222:dbl)  [unwired: 2 in, 2 out]
            n141 = case shown="1" w262 {
              tunnel: [1000.0 ("Value") 1.0 ("Value")] -> w261
              frame 0, Default {
              }
              frame 1 {
              }
            }
            n142 = case shown="2" w270 {
              tunnel: [1000000.0 ("Value") 1000.0 ("Value") 1.0 ("Value")] -> w272
              frame 0, Default {
              }
              frame 1 {
              }
              frame 2 {
              }
            }
            n143 = case shown="1" w276 {
              tunnel: [1000.0 ("Value") 1.0 ("Value")] -> w278
              frame 0, Default {
              }
              frame 1 {
              }
            }
            n144 = case shown="1" w273 {
              tunnel: [1000.0 ("Value") 1.0 ("Value")] -> w275
              frame 0, Default {
              }
              frame 1 {
              }
            }
            n145 = case shown="1" w281 {
              tunnel: [1000.0 ("Value") 1.0 ("Value")] -> w279
              frame 0, Default {
              }
              frame 1 {
              }
            }
            n146 = case shown="2" w219 {
              tunnel: [1000000.0 ("Value") 1000.0 ("Value") 1.0 ("Value")] -> w220
              frame 0, Default {
              }
              frame 1 {
              }
              frame 2 {
              }
            }
            n147 = case shown="1" w216 {
              tunnel: [1000.0 ("Value") 1.0 ("Value")] -> w215
              frame 0, Default {
              }
              frame 1 {
              }
            }
            n148 = case shown="0, 默认" w245 {
              tunnel: [Channel."Channel A" ("Channel (Channel A)") Channel."Channel B" ("Channel (Channel A)")] -> w224
              tunnel: ["smub" ("Script") "smua" ("Script")] -> w255
              frame 0, Default {
              }
              frame 1 {
              }
            }
            n149 = Divide(x=w260, y=w261) -> (x/y=w264:dbl)
            n150 = Divide(x=w277, y=w278) -> (x/y=w258:dbl)
            n151 = Divide(x=w274, y=w275) -> (x/y=w257:dbl)
            n152 = Divide(x=w280, y=w279) -> (x/y=w259:dbl)
            n153 = Divide(x=w271, y=w272) -> (x/y=w266:dbl)
            n154 = Divide(x=w222, y=w215) -> (x/y=w221:dbl)
            n155 = Divide(x=w218, y=w220) -> (x/y=w217:dbl)
            n156 = Number To Engineering String(2:w263, 4:w266) -> (0:w265:string)  [unwired: 2 in]
            n157 = Number To Engineering String(2:w263, 4:w259) -> (0:w254:string)  [unwired: 2 in]
            n158 = Number To Engineering String(2:w263, 4:w264) -> (0:w252:string)  [unwired: 2 in]
            n159 = Number To Engineering String(2:w263, 4:w258) -> (0:w253:string)  [unwired: 2 in]
            n160 = Number To Engineering String(2:w263, 4:w257) -> ()  [unwired: 2 in, 1 out]
            n161 = call <instrlib>:"Source Function.vi"("Function (Current)"=w231, "Channel (Channel A)"=w224, "Node In"=w223, "VISA resource name"=w227) -> ("error out"=w230:errorcluster, "Node Out"=w232:string, "VISA resource name out"=w233:refnum<visa-resource-name>)  [unwired: 1 in, 4 out]
            n162 = call "Keithley Sample Number.vi"("Step"=w257, "Stop"=w258, "Start"=w259) -> ("Array"=w236:dbl[], "pointnumber"=w250:dbl)  [unwired: 7 in]
            n163 = call <instrlib>:"Source Level.vi"("Level (0.000)"=w221, "Function (Current)"=w231, "error in (no error)"=w230, "Channel (Channel A)"=w224, "Node In"=w232, "VISA resource name"=w233) -> ("error out"=w229:errorcluster, "Node Out"=w235:string, "VISA resource name out"=w234:refnum<visa-resource-name>)  [unwired: 3 out]
            n164 = Number To Engineering String(2:i16 3 ("precision (6)"), 4:w250) -> (0:w248:string)  [unwired: 2 in]
            n165 = call <instrlib>:"Source Limit.vi"("Limit (0.000)"=w217, "Function (Current)"=enum32{"Current", "Voltage"}."Current", "error in (no error)"=w229, "Node In"=w235, "VISA resource name"=w234) -> ("error out"=w225:errorcluster, "VISA resource name out"=w226:refnum<visa-resource-name>)  [unwired: 1 in, 4 out]
            n166 = Concatenate Strings(w255, ".reset()\n" ("string"), w255, ".source.limiti=" ("string"), w265, "\nSweepILinMeasureI(" ("string"), w255, w247, w254, w247, w253, w247, w252, w247, w248, ")\nprintbuffer(1, " ("string"), w248, w247, ".nvbuffer1.readings)" ("string")) -> ()  [unwired: 1 out]
            n167 = call <instrlib>:"KE26XX Factory Pulse Script Usage.vi"("error in"=w225, "VISA resource name"=w226) -> ("Buffer Data"=w269:string)  [unwired: 8 in, 1 out]
            n168 = call <instrlib>:"Real 32 Converter.vi"("Data In"=w269) -> ("Data Array Out"=w237:sgl[])  [unwired: 10 in]
            n169 = for {
              tunnel: w236 -> [w291] mode=indexing
              tunnel: w237 -> [w289] mode=indexing
              tunnel: [w290] -> w240 mode=indexing
              tunnel: [w287] -> w239 mode=indexing
              w288 = i16 3 ("precision (6)")
              n170 = Number To Engineering String(2:w288, 4:w291) -> (0:w290:string)  [unwired: 2 in]
              n171 = Number To Engineering String(2:w288, 4:w289) -> (0:w287:string)  [unwired: 2 in]
            }
            n172 = Bundle("Array"=w236, "Data Array Out"=w237) -> (w243:cluster{"Array":dbl[], "Data Array Out":sgl[]})  [unwired: 1 in]
            n173 = Build Array (concatenate)(cluster{dbl[], dbl[]}[] [] ("Chart GL"), w243) -> (w242:cluster{"Array":dbl[], "Data Array Out":dbl[]}[])
            n174 = Build Array(w240, w239) -> (w241:string[][])
            n175 = property on="Chart GL" class="XYGraph (严格)"("Value"=w242) -> ()  [unwired: 2 in, 2 out]
            n176 = Transpose 2D Array(2D array=w241) -> (transposed array=w238:string[][])
            n177 = property on="Sheet GL" class="Tbl (严格)"("Value"=w238) -> ()  [unwired: 2 in, 2 out]
          }
        }
      }
    }
    n178 = property on="stop" class="Bool (严格)"() -> ("Value"=w14:bool)  [unwired: 2 in, 2 out]
  }
  n179 = while {
    stop <- "stop" stop-if-true
    n180 = event shown="[2] \"Save Button\": 值改变" {
      selector: _ -> [_ _ _]
      dyn-events: _ -> [_ _ _]
      timeout: _ -> [_ _ _]
      event "OK Button": Value Change {
        n181 = event-data() -> ()  [unwired: 1 in, 6 out]
      }
      event "DrainCluster DFC.DrainStartUnit DFC", "DrainCluster DFC.DrainStopUnit  DFC", "DrainCluster DFC.DrainStepUnit DFC", "GateCluster DFC.GateStartUnit DFC", "GateCluster DFC.GateStopUnit DFC", "GateCluster DFC.GateStepUnit DFC", "Series 2600B", "DrainCluster DFC.DrainCompUnit DFC", "GateCluster DFC.GateComplUnit DFC", "DrainClusterTV.StartUnit DrainTV", "DrainClusterTV.StopUnit DrainTV", "DrainClusterTV.StepUnit DrainTV", "DrainClusterTV.CompUnit DrainTV", "GateCluster TV.StartUnit GateTV", "GateCluster TV.StopUnit GateTV", "GateCluster TV.StepUnit GateTV", "GateCluster TV.CompUnit GateTV", "GateCluster GL.StartUnit GateGL", "GateCluster GL.StopUnit GateGL", "GateCluster GL.StepUnit GateGL", "GateCluster GL.CompUnit GateGL", "DrainCluster Trans.StartUnit DrainTR", "DrainCluster Trans.CompUnit DrainTR", "GateCluster Trans.StartUnit GateTR", "GateCluster Trans.StopUnit GateTR", "GateCluster Trans.StepUnit GateTR", "GateCluster Trans.CompUnit GateTR": Value Change {
        w309 = 0.01 ("Data Entry Limits:Minimum")
        w357 = 0.01 ("Data Entry Limits:Minimum")
        n182 = event-data() -> ()  [unwired: 1 in, 6 out]
        n183 = property on="Series 2600B" class="Ring (严格)"() -> ("Value"=w342:u16)  [unwired: 2 in, 2 out]
        n184 = property on="CompUnit DrainTR" class="Ring (严格)"() -> ("Value"=w359:u16)  [unwired: 2 in, 2 out]
        n185 = property on="CompUnit GateTR" class="Ring (严格)"() -> ("Value"=w358:u16)  [unwired: 2 in, 2 out]
        n186 = property on="DrainStopUnit  DFC" class="Ring (严格)"() -> ("Value"=w365:u16)  [unwired: 2 in, 2 out]
        n187 = property on="StartUnit GateTR" class="Ring (严格)"() -> ("Value"=w354:u16)  [unwired: 2 in, 2 out]
        n188 = property on="StopUnit GateTR" class="Ring (严格)"() -> ("Value"=w353:u16)  [unwired: 2 in, 2 out]
        n189 = property on="GateStartUnit DFC" class="Ring (严格)"() -> ("Value"=w379:u16)  [unwired: 2 in, 2 out]
        n190 = property on="GateStopUnit DFC" class="Ring (严格)"() -> ("Value"=w378:u16)  [unwired: 2 in, 2 out]
        n191 = property on="GateStepUnit DFC" class="Ring (严格)"() -> ("Value"=w367:u16)  [unwired: 2 in, 2 out]
        n192 = property on="DrainStartUnit DFC" class="Ring (严格)"() -> ("Value"=w366:u16)  [unwired: 2 in, 2 out]
        n193 = property on="DrainCompUnit DFC" class="Ring (严格)"() -> ("Value"=w361:u16)  [unwired: 2 in, 2 out]
        n194 = property on="GateComplUnit DFC" class="Ring (严格)"() -> ("Value"=w360:u16)  [unwired: 2 in, 2 out]
        n195 = property on="DrainStepUnit DFC" class="Ring (严格)"() -> ("Value"=w364:u16)  [unwired: 2 in, 2 out]
        n196 = property on="StepUnit GateTR" class="Ring (严格)"() -> ("Value"=w352:u16)  [unwired: 2 in, 2 out]
        n197 = property on="StartUnit DrainTR" class="Ring (严格)"() -> ("Value"=w351:u16)  [unwired: 2 in, 2 out]
        n198 = case shown="3..8" w342 {
          tunnel: [w505 w561] -> w380
          tunnel: [w493 w548] -> w363
          tunnel: w379 -> [w504 w560]
          tunnel: w378 -> [w503 w559]
          tunnel: [w502 w558] -> w376
          tunnel: [w501 w557] -> w375
          tunnel: [w500 w556] -> w373
          tunnel: [w499 w555] -> w371
          tunnel: [w498 w554] -> w368
          tunnel: w367 -> [w497 w553]
          tunnel: w366 -> [w496 w552]
          tunnel: w365 -> [w495 w551]
          tunnel: w364 -> [w494 w550]
          tunnel: w360 -> [w490 w547]
          tunnel: w361 -> [w492 w549]
          tunnel: [w491 w546] -> w362
          tunnel: w359 -> [w489 w544]
          tunnel: w358 -> [w488 w543]
          tunnel: [w487 w545] -> w356
          tunnel: [w486 w542] -> w355
          tunnel: w354 -> [w485 w541]
          tunnel: w353 -> [w484 w539]
          tunnel: w352 -> [w483 w537]
          tunnel: w351 -> [w482 w535]
          tunnel: [w481 w540] -> w350
          tunnel: [w480 w538] -> w347
          tunnel: [w479 w536] -> w345
          tunnel: [w478 w534] -> w343
          frame 0..2, Default {
            n199 = case shown="2" w492 {
              tunnel: [900.0 ("Data Entry Limits:Maximum") 10.0 ("Data Entry Limits:Maximum")] -> w493
              frame 0, 1, Default {
              }
              frame 2 {
              }
            }
            n200 = case shown="1" w496 {
              tunnel: [900.0 ("Data Entry Limits:Maximum") 40.0 ("Data Entry Limits:Maximum")] -> w500
              frame 0, Default {
              }
              frame 1 {
              }
            }
            n201 = case shown="1" w495 {
              tunnel: [900.0 ("Data Entry Limits:Maximum") 40.0 ("Data Entry Limits:Maximum")] -> w499
              frame 0, Default {
              }
              frame 1 {
              }
            }
            n202 = case shown="1" w497 {
              tunnel: [900.0 ("Data Entry Limits:Maximum") 40.0 ("Data Entry Limits:Maximum")] -> w501
              frame 0, Default {
              }
              frame 1 {
              }
            }
            n203 = case shown="1" w494 {
              tunnel: [900.0 ("Data Entry Limits:Maximum") 40.0 ("Data Entry Limits:Maximum")] -> w498
              frame 0, Default {
              }
              frame 1 {
              }
            }
            n204 = case shown="2" w490 {
              tunnel: [900.0 ("Data Entry Limits:Maximum") 10.0 ("Data Entry Limits:Maximum")] -> w491
              frame 0, 1, Default {
              }
              frame 2 {
              }
            }
            n205 = case shown="1" w503 {
              tunnel: [900.0 ("Data Entry Limits:Maximum") 40.0 ("Data Entry Limits:Maximum")] -> w502
              frame 0, Default {
              }
              frame 1 {
              }
            }
            n206 = case shown="2" w488 {
              tunnel: [900.0 ("Data Entry Limits:Maximum") 10.0 ("Data Entry Limits:Maximum")] -> w486
              frame 0, 1, Default {
              }
              frame 2 {
              }
            }
            n207 = case shown="1" w482 {
              tunnel: [900.0 ("Data Entry Limits:Maximum") 40.0 ("Data Entry Limits:Maximum")] -> w478
              frame 0, Default {
              }
              frame 1 {
              }
            }
            n208 = case shown="1" w504 {
              tunnel: [900.0 ("Data Entry Limits:Maximum") 40.0 ("Data Entry Limits:Maximum")] -> w505
              frame 0, Default {
              }
              frame 1 {
              }
            }
            n209 = case shown="1" w483 {
              tunnel: [900.0 ("Data Entry Limits:Maximum") 40.0 ("Data Entry Limits:Maximum")] -> w479
              frame 0, Default {
              }
              frame 1 {
              }
            }
            n210 = case shown="1" w484 {
              tunnel: [900.0 ("Data Entry Limits:Maximum") 40.0 ("Data Entry Limits:Maximum")] -> w480
              frame 0, Default {
              }
              frame 1 {
              }
            }
            n211 = case shown="2" w489 {
              tunnel: [900.0 ("Data Entry Limits:Maximum") 10.0 ("Data Entry Limits:Maximum")] -> w487
              frame 0, 1, Default {
              }
              frame 2 {
              }
            }
            n212 = case shown="1" w485 {
              tunnel: [900.0 ("Data Entry Limits:Maximum") 40.0 ("Data Entry Limits:Maximum")] -> w481
              frame 0, Default {
              }
              frame 1 {
              }
            }
          }
          frame 3..8 {
            n213 = case shown="0, 默认" w537 {
              tunnel: [900.0 ("Data Entry Limits:Maximum") 200.0 ("Data Entry Limits:Maximum")] -> w536
              frame 0, Default {
              }
              frame 1 {
              }
            }
            n214 = case shown="0, 默认" w551 {
              tunnel: [900.0 ("Data Entry Limits:Maximum") 200.0 ("Data Entry Limits:Maximum")] -> w555
              frame 0, Default {
              }
              frame 1 {
              }
            }
            n215 = case shown="0, 默认" w535 {
              tunnel: [900.0 ("Data Entry Limits:Maximum") 200.0 ("Data Entry Limits:Maximum")] -> w534
              frame 0, Default {
              }
              frame 1 {
              }
            }
            n216 = case shown="1" w560 {
              tunnel: [900.0 ("Data Entry Limits:Maximum") 200.0 ("Data Entry Limits:Maximum")] -> w561
              frame 0, Default {
              }
              frame 1 {
              }
            }
            n217 = case shown="0, 默认" w553 {
              tunnel: [900.0 ("Data Entry Limits:Maximum") 200.0 ("Data Entry Limits:Maximum")] -> w557
              frame 0, Default {
              }
              frame 1 {
              }
            }
            n218 = case shown="0, 默认" w550 {
              tunnel: [900.0 ("Data Entry Limits:Maximum") 200.0 ("Data Entry Limits:Maximum")] -> w554
              frame 0, Default {
              }
              frame 1 {
              }
            }
            n219 = case shown="2" w549 {
              tunnel: [900.0 ("Data Entry Limits:Maximum") 10.0 ("Data Entry Limits:Maximum")] -> w548
              frame 0, 1, Default {
              }
              frame 2 {
              }
            }
            n220 = case shown="2" w547 {
              tunnel: [900.0 ("Data Entry Limits:Maximum") 10.0 ("Data Entry Limits:Maximum")] -> w546
              frame 0, 1, Default {
              }
              frame 2 {
              }
            }
            n221 = case shown="0, 默认" w539 {
              tunnel: [900.0 ("Data Entry Limits:Maximum") 200.0 ("Data Entry Limits:Maximum")] -> w538
              frame 0, Default {
              }
              frame 1 {
              }
            }
            n222 = case shown="0, 默认" w559 {
              tunnel: [900.0 ("Data Entry Limits:Maximum") 200.0 ("Data Entry Limits:Maximum")] -> w558
              frame 0, Default {
              }
              frame 1 {
              }
            }
            n223 = case shown="0, 默认" w552 {
              tunnel: [900.0 ("Data Entry Limits:Maximum") 200.0 ("Data Entry Limits:Maximum")] -> w556
              frame 0, Default {
              }
              frame 1 {
              }
            }
            n224 = case shown="2" w543 {
              tunnel: [900.0 ("Data Entry Limits:Maximum") 10.0 ("Data Entry Limits:Maximum")] -> w542
              frame 0, 1, Default {
              }
              frame 2 {
              }
            }
            n225 = case shown="2" w544 {
              tunnel: [900.0 ("Data Entry Limits:Maximum") 10.0 ("Data Entry Limits:Maximum")] -> w545
              frame 0, 1, Default {
              }
              frame 2 {
              }
            }
            n226 = case shown="0, 默认" w541 {
              tunnel: [900.0 ("Data Entry Limits:Maximum") 200.0 ("Data Entry Limits:Maximum")] -> w540
              frame 0, Default {
              }
              frame 1 {
              }
            }
          }
        }
        n227 = Negate(x=w350) -> (-x=w349:dbl)
        n228 = Negate(x=w345) -> (-x=w346:dbl)
        n229 = Negate(x=w380) -> (-x=w381:dbl)
        n230 = Negate(x=w376) -> (-x=w377:dbl)
        n231 = Negate(x=w375) -> (-x=w374:dbl)
        n232 = Negate(x=w373) -> (-x=w372:dbl)
        n233 = Negate(x=w371) -> (-x=w370:dbl)
        n234 = Negate(x=w368) -> (-x=w369:dbl)
        n235 = Negate(x=w343) -> (-x=w344:dbl)
        n236 = property on="Step GateTR" class="DigNum (严格)"("Maximum"=w345, "Minimum"=w346) -> ()  [unwired: 2 in, 2 out]
        n237 = property on="Start  GateTR" class="DigNum (严格)"("Maximum"=w350, "Minimum"=w349) -> ()  [unwired: 2 in, 2 out]
        n238 = property on="Comp DrainTR" class="DigNum (严格)"("Maximum"=w356, "Minimum"=w357) -> ()  [unwired: 2 in, 2 out]
        n239 = property on="GateComp DFC" class="DigNum (严格)"("Maximum"=w362, "Minimum"=w357) -> ()  [unwired: 2 in, 2 out]
        n240 = property on="GateStart DFC" class="DigNum (严格)"("Maximum"=w380, "Minimum"=w381) -> ()  [unwired: 2 in, 2 out]
        n241 = property on="GateStopDFC" class="DigNum (严格)"("Maximum"=w376, "Minimum"=w377) -> ()  [unwired: 2 in, 2 out]
        n242 = property on="GateStepDFC" class="DigNum (严格)"("Maximum"=w375, "Minimum"=w374) -> ()  [unwired: 2 in, 2 out]
        n243 = property on="DrainStart DFC" class="DigNum (严格)"("Maximum"=w373, "Minimum"=w372) -> ()  [unwired: 2 in, 2 out]
        n244 = property on="DrainStop DFC" class="DigNum (严格)"("Maximum"=w371, "Minimum"=w370) -> ()  [unwired: 2 in, 2 out]
        n245 = property on="DrainStep DFC" class="DigNum (严格)"("Maximum"=w368, "Minimum"=w369) -> ()  [unwired: 2 in, 2 out]
        n246 = property on="DrainComp DFC" class="DigNum (严格)"("Maximum"=w363, "Minimum"=w357) -> ()  [unwired: 2 in, 2 out]
        n247 = Negate(x=w347) -> (-x=w348:dbl)
        n248 = property on="Start DrainTR" class="DigNum (严格)"("Maximum"=w343, "Minimum"=w344) -> ()  [unwired: 2 in, 2 out]
        n249 = property on="Stop GateTR" class="DigNum (严格)"("Maximum"=w347, "Minimum"=w348) -> ()  [unwired: 2 in, 2 out]
        n250 = property on="Comp GateTR" class="DigNum (严格)"("Maximum"=w355, "Minimum"=w357) -> ()  [unwired: 2 in, 2 out]
        n251 = property on="StopUnit GateGL" class="Ring (严格)"() -> ("Value"=w336:u16)  [unwired: 2 in, 2 out]
        n252 = property on="StepUnit GateGL" class="Ring (严格)"() -> ("Value"=w333:u16)  [unwired: 2 in, 2 out]
        n253 = property on="StartUnit GateTV" class="Ring (严格)"() -> ("Value"=w329:u16)  [unwired: 2 in, 2 out]
        n254 = property on="StartUnit GateGL" class="Ring (严格)"() -> ("Value"=w339:u16)  [unwired: 2 in, 2 out]
        n255 = property on="StopUnit GateTV" class="Ring (严格)"() -> ("Value"=w326:u16)  [unwired: 2 in, 2 out]
        n256 = property on="StepUnit GateTV" class="Ring (严格)"() -> ("Value"=w323:u16)  [unwired: 2 in, 2 out]
        n257 = property on="CompUnit GateTV" class="Ring (严格)"() -> ("Value"=w310:u16)  [unwired: 2 in, 2 out]
        n258 = property on="StopUnit DrainTV" class="Ring (严格)"() -> ("Value"=w317:u16)  [unwired: 2 in, 2 out]
        n259 = property on="StepUnit DrainTV" class="Ring (严格)"() -> ("Value"=w318:u16)  [unwired: 2 in, 2 out]
        n260 = property on="CompUnit DrainTV" class="Ring (严格)"() -> ("Value"=w330:u16)  [unwired: 2 in, 2 out]
        n261 = property on="StartUnit DrainTV" class="Ring (严格)"() -> ("Value"=w319:u16)  [unwired: 2 in, 2 out]
        n262 = property on="CompUnit GateGL" class="Ring (严格)"() -> ("Value"=w341:u16)  [unwired: 2 in, 2 out]
        n263 = case shown="0..2, 默认" w342 {
          tunnel: [w405 w453] -> w338
          tunnel: [w393 w440] -> w340
          tunnel: w339 -> [w404 w452]
          tunnel: w336 -> [w403 w451]
          tunnel: [w402 w450] -> w335
          tunnel: [w401 w449] -> w332
          tunnel: [w400 w448] -> w328
          tunnel: [w399 w447] -> w325
          tunnel: [w398 w446] -> w322
          tunnel: w333 -> [w397 w445]
          tunnel: w329 -> [w396 w444]
          tunnel: w326 -> [w395 w443]
          tunnel: w323 -> [w394 w442]
          tunnel: w330 -> [w390 w439]
          tunnel: w341 -> [w392 w441]
          tunnel: [w391 w438] -> w320
          tunnel: w319 -> [w382 w437]
          tunnel: w317 -> [w387 w435]
          tunnel: [w383 w436] -> w315
          tunnel: [w386 w434] -> w313
          tunnel: w318 -> [w389 w432]
          tunnel: [w388 w433] -> w312
          tunnel: w310 -> [w385 w431]
          tunnel: [w384 w430] -> w308
          frame 0..2, Default {
            n264 = case shown="2" w392 {
              tunnel: [900.0 ("Data Entry Limits:Maximum") 10.0 ("Data Entry Limits:Maximum")] -> w393
              frame 0, 1, Default {
              }
              frame 2 {
              }
            }
            n265 = case shown="1" w396 {
              tunnel: [900.0 ("Data Entry Limits:Maximum") 40.0 ("Data Entry Limits:Maximum")] -> w400
              frame 0, Default {
              }
              frame 1 {
              }
            }
            n266 = case shown="1" w395 {
              tunnel: [900.0 ("Data Entry Limits:Maximum") 40.0 ("Data Entry Limits:Maximum")] -> w399
              frame 0, Default {
              }
              frame 1 {
              }
            }
            n267 = case shown="1" w397 {
              tunnel: [900.0 ("Data Entry Limits:Maximum") 40.0 ("Data Entry Limits:Maximum")] -> w401
              frame 0, Default {
              }
              frame 1 {
              }
            }
            n268 = case shown="1" w394 {
              tunnel: [900.0 ("Data Entry Limits:Maximum") 40.0 ("Data Entry Limits:Maximum")] -> w398
              frame 0, Default {
              }
              frame 1 {
              }
            }
            n269 = case shown="2" w390 {
              tunnel: [900.0 ("Data Entry Limits:Maximum") 10.0 ("Data Entry Limits:Maximum")] -> w391
              frame 0, 1, Default {
              }
              frame 2 {
              }
            }
            n270 = case shown="1" w403 {
              tunnel: [900.0 ("Data Entry Limits:Maximum") 40.0 ("Data Entry Limits:Maximum")] -> w402
              frame 0, Default {
              }
              frame 1 {
              }
            }
            n271 = case shown="2" w385 {
              tunnel: [900.0 ("Data Entry Limits:Maximum") 10.0 ("Data Entry Limits:Maximum")] -> w384
              frame 0, 1, Default {
              }
              frame 2 {
              }
            }
            n272 = case shown="1" w382 {
              tunnel: [900.0 ("Data Entry Limits:Maximum") 40.0 ("Data Entry Limits:Maximum")] -> w383
              frame 0, Default {
              }
              frame 1 {
              }
            }
            n273 = case shown="1" w404 {
              tunnel: [900.0 ("Data Entry Limits:Maximum") 40.0 ("Data Entry Limits:Maximum")] -> w405
              frame 0, Default {
              }
              frame 1 {
              }
            }
            n274 = case shown="1" w387 {
              tunnel: [900.0 ("Data Entry Limits:Maximum") 40.0 ("Data Entry Limits:Maximum")] -> w386
              frame 0, Default {
              }
              frame 1 {
              }
            }
            n275 = case shown="1" w389 {
              tunnel: [900.0 ("Data Entry Limits:Maximum") 40.0 ("Data Entry Limits:Maximum")] -> w388
              frame 0, Default {
              }
              frame 1 {
              }
            }
          }
          frame 3..8 {
            n276 = case shown="0, 默认" w443 {
              tunnel: [900.0 ("Data Entry Limits:Maximum") 200.0 ("Data Entry Limits:Maximum")] -> w447
              frame 0, Default {
              }
              frame 1 {
              }
            }
            n277 = case shown="1" w452 {
              tunnel: [900.0 ("Data Entry Limits:Maximum") 200.0 ("Data Entry Limits:Maximum")] -> w453
              frame 0, Default {
              }
              frame 1 {
              }
            }
            n278 = case shown="0, 默认" w445 {
              tunnel: [900.0 ("Data Entry Limits:Maximum") 200.0 ("Data Entry Limits:Maximum")] -> w449
              frame 0, Default {
              }
              frame 1 {
              }
            }
            n279 = case shown="0, 默认" w442 {
              tunnel: [900.0 ("Data Entry Limits:Maximum") 200.0 ("Data Entry Limits:Maximum")] -> w446
              frame 0, Default {
              }
              frame 1 {
              }
            }
            n280 = case shown="2" w441 {
              tunnel: [900.0 ("Data Entry Limits:Maximum") 10.0 ("Data Entry Limits:Maximum")] -> w440
              frame 0, 1, Default {
              }
              frame 2 {
              }
            }
            n281 = case shown="2" w439 {
              tunnel: [900.0 ("Data Entry Limits:Maximum") 10.0 ("Data Entry Limits:Maximum")] -> w438
              frame 0, 1, Default {
              }
              frame 2 {
              }
            }
            n282 = case shown="1" w451 {
              tunnel: [900.0 ("Data Entry Limits:Maximum") 200.0 ("Data Entry Limits:Maximum")] -> w450
              frame 0, Default {
              }
              frame 1 {
              }
            }
            n283 = case shown="0, 默认" w444 {
              tunnel: [900.0 ("Data Entry Limits:Maximum") 200.0 ("Data Entry Limits:Maximum")] -> w448
              frame 0, Default {
              }
              frame 1 {
              }
            }
            n284 = case shown="1" w437 {
              tunnel: [900.0 ("Data Entry Limits:Maximum") 200.0 ("Data Entry Limits:Maximum")] -> w436
              frame 0, Default {
              }
              frame 1 {
              }
            }
            n285 = case shown="1" w432 {
              tunnel: [900.0 ("Data Entry Limits:Maximum") 200.0 ("Data Entry Limits:Maximum")] -> w433
              frame 0, Default {
              }
              frame 1 {
              }
            }
            n286 = case shown="1" w435 {
              tunnel: [900.0 ("Data Entry Limits:Maximum") 200.0 ("Data Entry Limits:Maximum")] -> w434
              frame 0, Default {
              }
              frame 1 {
              }
            }
            n287 = case shown="2" w431 {
              tunnel: [900.0 ("Data Entry Limits:Maximum") 10.0 ("Data Entry Limits:Maximum")] -> w430
              frame 0, 1, Default {
              }
              frame 2 {
              }
            }
          }
        }
        n288 = Negate(x=w312) -> (-x=w311:dbl)
        n289 = Negate(x=w338) -> (-x=w337:dbl)
        n290 = Negate(x=w335) -> (-x=w334:dbl)
        n291 = Negate(x=w332) -> (-x=w331:dbl)
        n292 = Negate(x=w328) -> (-x=w327:dbl)
        n293 = Negate(x=w325) -> (-x=w324:dbl)
        n294 = Negate(x=w322) -> (-x=w321:dbl)
        n295 = Negate(x=w315) -> (-x=w316:dbl)
        n296 = Negate(x=w313) -> (-x=w314:dbl)
        n297 = property on="Start DrainTV" class="DigNum (严格)"("Maximum"=w315, "Minimum"=w316) -> ()  [unwired: 2 in, 2 out]
        n298 = property on="Start GateGL" class="DigNum (严格)"("Maximum"=w338, "Minimum"=w337) -> ()  [unwired: 2 in, 2 out]
        n299 = property on="Stop GateGL" class="DigNum (严格)"("Maximum"=w335, "Minimum"=w334) -> ()  [unwired: 2 in, 2 out]
        n300 = property on="Step GateGL" class="DigNum (严格)"("Maximum"=w332, "Minimum"=w331) -> ()  [unwired: 2 in, 2 out]
        n301 = property on="Start GateTV" class="DigNum (严格)"("Maximum"=w328, "Minimum"=w327) -> ()  [unwired: 2 in, 2 out]
        n302 = property on="Stop GateTV" class="DigNum (严格)"("Maximum"=w325, "Minimum"=w324) -> ()  [unwired: 2 in, 2 out]
        n303 = property on="Step GateTV" class="DigNum (严格)"("Maximum"=w322, "Minimum"=w321) -> ()  [unwired: 2 in, 2 out]
        n304 = property on="Comp DrainTV" class="DigNum (严格)"("Maximum"=w320, "Minimum"=w309) -> ()  [unwired: 2 in, 2 out]
        n305 = property on="Comp GateGL" class="DigNum (严格)"("Maximum"=w340, "Minimum"=w309) -> ()  [unwired: 2 in, 2 out]
        n306 = property on="Comp GateTV" class="DigNum (严格)"("Maximum"=w308, "Minimum"=w309) -> ()  [unwired: 2 in, 2 out]
        n307 = property on="Stop DrainTV" class="DigNum (严格)"("Maximum"=w313, "Minimum"=w314) -> ()  [unwired: 2 in, 2 out]
        n308 = property on="Step DrainTV" class="DigNum (严格)"("Maximum"=w312, "Minimum"=w311) -> ()  [unwired: 2 in, 2 out]
      }
      event "Save Button": Value Change {
        n309 = event-data() -> ("NewVal"=w590:bool)  [unwired: 1 in, 5 out]
        n310 = case shown="真" w590 {
          frame False {
          }
          frame True {
            n311 = property on="Tab Control" class="TabCtl (严格)"() -> ("Value"=w591:T1)  [unwired: 2 in, 2 out]
            n312 = case shown="\"Drain Family of Curves \", 默认" w591 {
              frame "Drain Family of Curves ", Default {
                n313 = property on="DrainStart DFC" class="DigNum (严格)"() -> ("Value"=w613:dbl)  [unwired: 2 in, 2 out]
                n314 = property on="DrainStep DFC" class="DigNum (严格)"() -> ("Value"=w593:dbl)  [unwired: 2 in, 2 out]
                n315 = property on="DrainStop DFC" class="DigNum (严格)"() -> ("Value"=w594:dbl)  [unwired: 2 in, 2 out]
                n316 = property on="DrainStartUnit DFC" class="Ring (严格)"() -> ("Value"=w612:u16)  [unwired: 2 in, 2 out]
                n317 = property on="DrainStopUnit  DFC" class="Ring (严格)"() -> ("Value"=w610:u16)  [unwired: 2 in, 2 out]
                n318 = Number To Fractional String(number=w594) -> (F-format string=w604:string)  [unwired: 3 in]
                n319 = Number To Fractional String(number=w593) -> (F-format string=w603:string)  [unwired: 3 in]
                n320 = Number To Fractional String(number=w613) -> (F-format string=w605:string)  [unwired: 3 in]
                n321 = case shown="1" w610 {
                  tunnel: ["mV" "V"] -> w598
                  frame 0, Default {
                  }
                  frame 1 {
                  }
                }
                n322 = case shown="1" w612 {
                  tunnel: ["mV" "V"] -> w599
                  frame 0, Default {
                  }
                  frame 1 {
                  }
                }
                n323 = call "StringClearZero.vi"("String in"=w603) -> ("String out"=w601:string)  [unwired: 10 in]
                n324 = call "StringClearZero.vi"("String in"=w604) -> ("String out"=w600:string)  [unwired: 10 in]
                n325 = call "StringClearZero.vi"("String in"=w605) -> ("String out"=w602:string)  [unwired: 10 in]
                n326 = property on="DrainStepUnit DFC" class="Ring (严格)"() -> ("Value"=w611:u16)  [unwired: 2 in, 2 out]
                n327 = property on="DrainComp DFC" class="DigNum (严格)"() -> ("Value"=w609:dbl)  [unwired: 2 in, 2 out]
                n328 = property on="DrainCompUnit DFC" class="Ring (严格)"() -> ("Value"=w596:u16)  [unwired: 2 in, 2 out]
                n329 = case shown="0, 默认" w611 {
                  tunnel: [" mV" "V"] -> w597
                  frame 0, Default {
                  }
                  frame 1 {
                  }
                }
                n330 = Number To Fractional String(number=w609) -> (F-format string=w608:string)  [unwired: 3 in]
                n331 = case shown="2" w596 {
                  tunnel: ["μA" "mA" "A"] -> w595
                  frame 0, Default {
                  }
                  frame 1 {
                  }
                  frame 2 {
                  }
                }
                n332 = property on="Sheet DFC" class="Tbl (严格)"() -> ("Value"=w606:string[][])  [unwired: 2 in, 2 out]
                n333 = Get Date/Time In Seconds() -> (seconds since 1Jan1904=w592:timestamp)
                n334 = call "Keithley Report2400.vi"("Test operator"="深圳市展芯科技有限公司", "Start"=w602, "Stop"=w600, "Step"=w601, "Compliance"=w608, "Data"=w606, "Comp Unit"=w595, "Start unit"=w599, "test time"=w592, "Stop Unit"=w598, "StepUnit"=w597) -> ()  [unwired: 9 in]
              }
              frame "Threshold Voltage" {
              }
              frame "Gate Leakage" {
              }
              frame "Transconductance" {
              }
            }
          }
        }
      }
    }
  }
